vi "Test Serializer.Text.issue5.vi"(8 "error in (no error)":errorcluster) -> (0 "error out":errorcluster)   [LabVIEW 2013]
uses:
  source/Serializer.PlainText/Serializer.PlainText.lvclass
  <vilib>/addons/_JKI Toolkits/Caraya/classes/Assert/Assert Not Error.vi
  <vilib>/addons/_JKI Toolkits/Caraya/classes/Assert/Assert Equal Value and Type_Variant.vi
  <vilib>/addons/_JKI Toolkits/Caraya/classes/Assert/Assert.lvclass
  source/Serializer/Serializer.lvclass
  <vilib>/addons/_JKI Toolkits/Caraya/classes/Test/Test.lvclass
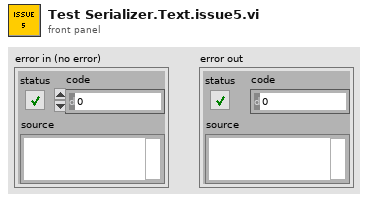
[diagram p1: front panel]
types:
  T1 = cluster{"String":string, "Cluster Array":cluster{"String":string, "Number":i16}[]}
  T2 = cluster{"String":string, "Cluster 2":cluster{"String":string, "Number":i16}}[]
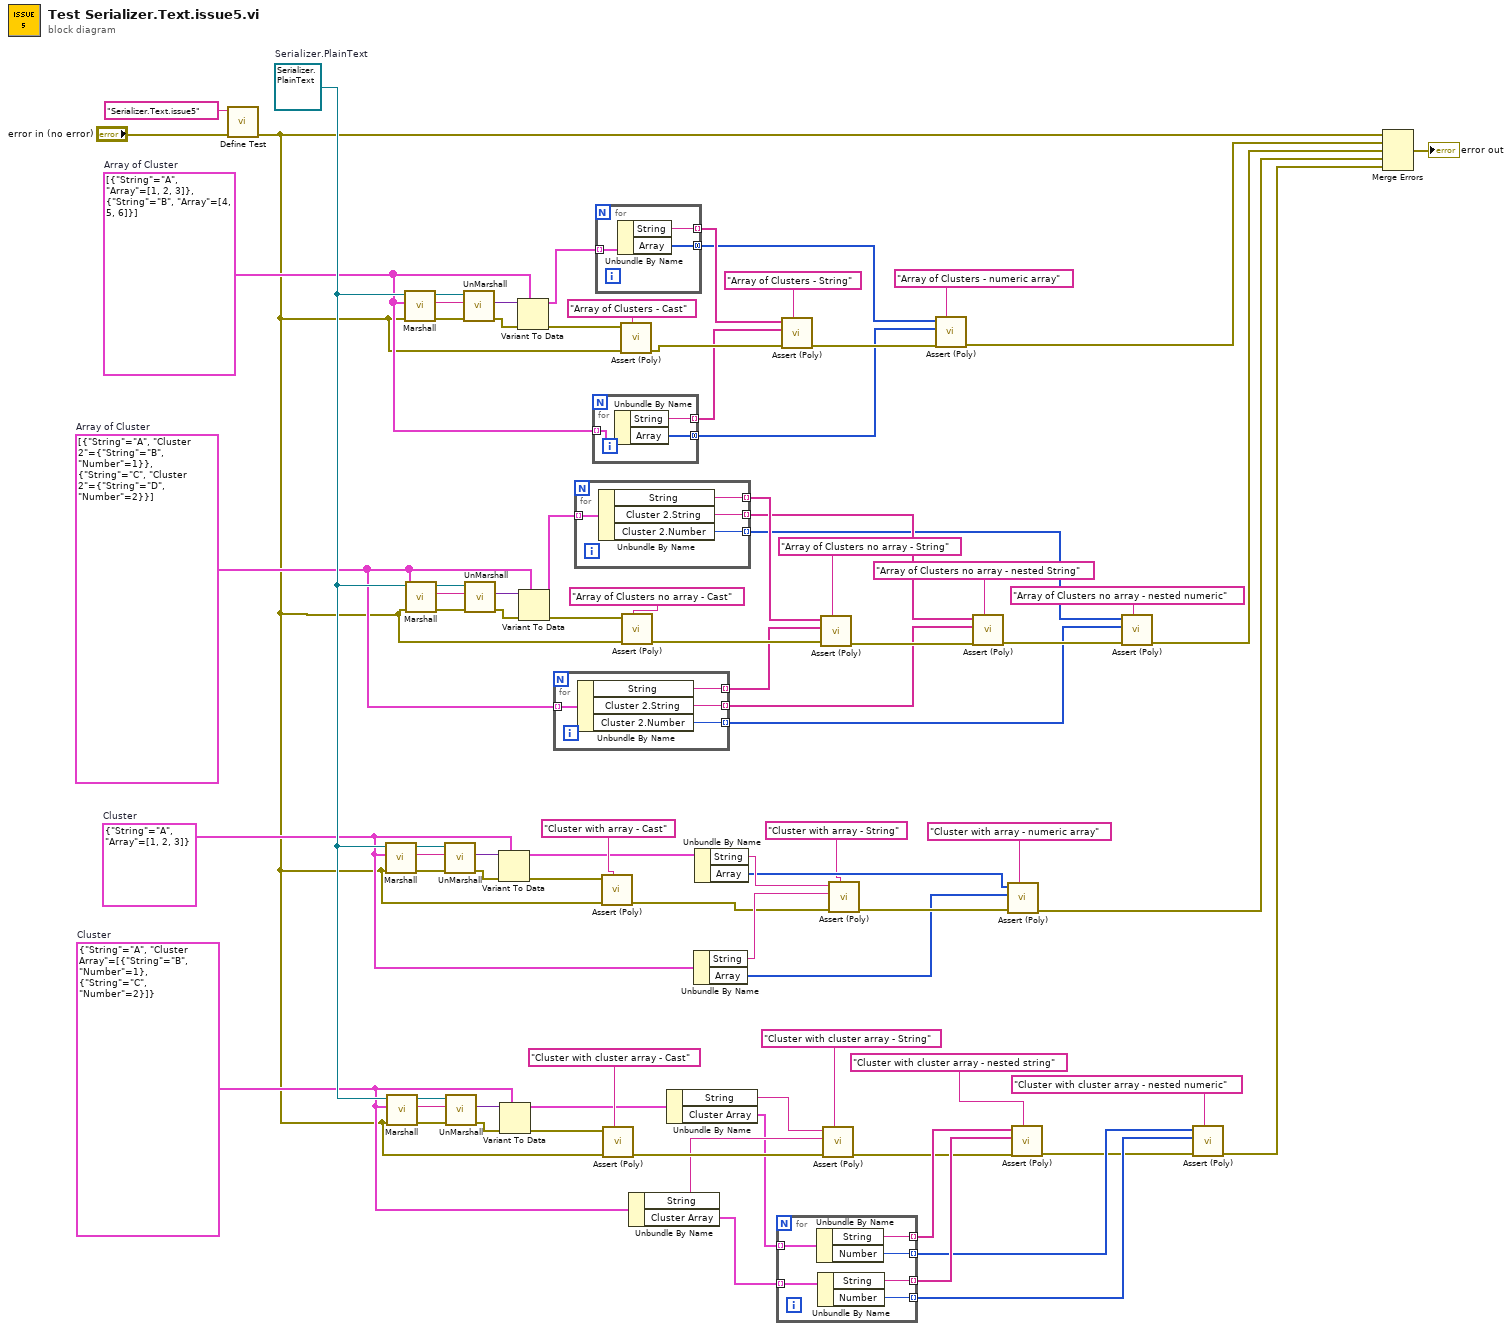
[diagram p0: block diagram]
diagram:
  w18 = T1 {"String"="A", "Cluster Array"=[{"String"="B", "Number"=1}, {"String"="C", "Number"=2}]}  # Cluster
  w31 = cluster{"String":string, "Array":i16[]} {"String"="A", "Array"=[1, 2, 3]}  # Cluster
  w3 = T2 [{"String"="A", "Cluster 2"={"String"="B", "Number"=1}}, {"String"="C", "Cluster 2"={"String"="D", "Number"=2}}]  # Array of Cluster
  w4 = cluster{"String":string, "Array":i16[]}[] [{"String"="A", "Array"=[1, 2, 3]}, {"String"="B", "Array"=[4, 5, 6]}]  # Array of Cluster
  w57 = refnum<class "Serializer.PlainText.lvclass"> refnum  # Serializer.PlainText
  n1 = call <vilib>:"Define Test.vi"("error in (no error)"="error in (no error)", "Label (VI Title)"="Serializer.Text.issue5") -> ("error out"=w1:errorcluster)  [unwired: 9 in]
  n2 = call "Marshall.vi"("error in (no error)"=w1, "Variant"=w31, "Serializer in"=w57) -> ("error out"=w70:errorcluster, "String"=w72:string, "Serializer out"=w71:refnum<class "Serializer.PlainText.lvclass">)  [unwired: 6 in]
  n3 = call "Marshall.vi"("error in (no error)"=w1, "Variant"=w18, "Serializer in"=w57) -> ("error out"=w61:errorcluster, "String"=w59:string, "Serializer out"=w60:refnum<class "Serializer.PlainText.lvclass">)  [unwired: 6 in]
  n4 = call "Marshall.vi"("error in (no error)"=w1, "Variant"=w4, "Serializer in"=w57) -> ("error out"=w82:errorcluster, "String"=w84:string, "Serializer out"=w83:refnum<class "Serializer.PlainText.lvclass">)  [unwired: 6 in]
  n5 = call "Marshall.vi"("error in (no error)"=w1, "Variant"=w3, "Serializer in"=w57) -> ("error out"=w77:errorcluster, "String"=w75:string, "Serializer out"=w76:refnum<class "Serializer.PlainText.lvclass">)  [unwired: 6 in]
  n6 = call "UnMarshall.vi"("error in (no error)"=w70, "String"=w72, "Serializer in"=w71) -> ("error out"=w65:errorcluster, "Variant"=w69:variant)  [unwired: 6 in, 1 out]
  n7 = call "UnMarshall.vi"("error in (no error)"=w61, "String"=w59, "Serializer in"=w60) -> ("error out"=w64:errorcluster, "Variant"=w62:variant)  [unwired: 6 in, 1 out]
  n8 = call "UnMarshall.vi"("error in (no error)"=w82, "String"=w84, "Serializer in"=w83) -> ("error out"=w67:errorcluster, "Variant"=w81:variant)  [unwired: 6 in, 1 out]
  n9 = call "UnMarshall.vi"("error in (no error)"=w77, "String"=w75, "Serializer in"=w76) -> ("error out"=w66:errorcluster, "Variant"=w78:variant)  [unwired: 6 in, 1 out]
  n10 = Variant To Data(error in=w65, type=w31, Variant=w69) -> (data=w32:cluster{"String":string, "Array":i16[]}, error out=w68:errorcluster)
  n11 = Variant To Data(error in=w64, type=w18, Variant=w62) -> (data=w19:T1, error out=w63:errorcluster)
  n12 = Variant To Data(error in=w67, type=w4, Variant=w81) -> (data=w51:cluster{"String":string, "Array":i16[]}[], error out=w80:errorcluster)
  n13 = Variant To Data(error in=w66, type=w3, Variant=w78) -> (data=w50:T2, error out=w79:errorcluster)
  n14 = for {
    tunnel: w3 -> [w91] mode=indexing
    tunnel: [w90] -> w37 mode=indexing
    tunnel: [w89] -> w35 mode=indexing
    tunnel: [w88] -> w33 mode=indexing
    n15 = Unbundle By Name(w91) -> ("String"=w90:string, "Cluster 2.String"=w89:string, "Cluster 2.Number"=w88:i16)
  }
  n16 = for {
    tunnel: w50 -> [w95] mode=indexing
    tunnel: [w94] -> w38 mode=indexing
    tunnel: [w93] -> w36 mode=indexing
    tunnel: [w92] -> w34 mode=indexing
    n17 = Unbundle By Name(w95) -> ("String"=w94:string, "Cluster 2.String"=w93:string, "Cluster 2.Number"=w92:i16)
  }
  n18 = for {
    tunnel: [w98] -> w47 mode=concatenating
    tunnel: [w97] -> w48 mode=indexing
    tunnel: w4 -> [w96] mode=indexing
    n19 = Unbundle By Name(w96) -> ("String"=w97:string, "Array"=w98:i16[])
  }
  n20 = for {
    tunnel: w51 -> [w101] mode=indexing
    tunnel: [w100] -> w46 mode=concatenating
    tunnel: [w99] -> w49 mode=indexing
    n21 = Unbundle By Name(w101) -> ("String"=w99:string, "Array"=w100:i16[])
  }
  n22 = call-poly <vilib>:"Assert (Poly).vi"("Label"="Cluster with array - Cast", "error in (no error)"=w1, "Not Error?"=w68) -> ("error out"=w28:errorcluster)  [unwired: 8 in]
  n23 = call-poly <vilib>:"Assert (Poly).vi"("Label"="Cluster with cluster array - Cast", "error in (no error)"=w1, "Not Error?"=w63) -> ("error out"=w21:errorcluster)  [unwired: 8 in]
  n24 = call-poly <vilib>:"Assert (Poly).vi"("Label"="Array of Clusters - Cast", "error in (no error)"=w1, "Not Error?"=w80) -> ("error out"=w56:errorcluster)  [unwired: 8 in]
  n25 = call-poly <vilib>:"Assert (Poly).vi"("Label"="Array of Clusters no array - Cast", "error in (no error)"=w1, "Not Error?"=w79) -> ("error out"=w42:errorcluster)  [unwired: 8 in]
  n26 = Unbundle By Name(w18) -> ("String"=w14:string, "Cluster Array"=w13:cluster{"String":string, "Number":i16}[])
  n27 = Unbundle By Name(w19) -> ("String"=w15:string, "Cluster Array"=w12:cluster{"String":string, "Number":i16}[])
  n28 = Unbundle By Name(w31) -> ("String"=w29:string, "Array"=w25:i16[])
  n29 = Unbundle By Name(w32) -> ("String"=w30:string, "Array"=w26:i16[])
  n30 = for {
    tunnel: w13 -> [w106] mode=indexing
    tunnel: w12 -> [w107] mode=indexing
    tunnel: [w105] -> w11 mode=indexing
    tunnel: [w104] -> w9 mode=indexing
    tunnel: [w103] -> w10 mode=indexing
    tunnel: [w102] -> w8 mode=indexing
    n31 = Unbundle By Name(w107) -> ("String"=w105:string, "Number"=w104:i16)
    n32 = Unbundle By Name(w106) -> ("String"=w103:string, "Number"=w102:i16)
  }
  n33 = call-poly <vilib>:"Assert (Poly).vi"("Label"="Array of Clusters - String", "error in (no error)"=w56, "Y"=w48, "X"=w49) -> ("error out"=w55:errorcluster)  [unwired: 7 in]
  n34 = call-poly <vilib>:"Assert (Poly).vi"("Label"="Array of Clusters no array - String", "error in (no error)"=w42, "Y"=w37, "X"=w38) -> ("error out"=w41:errorcluster)  [unwired: 7 in]
  n35 = call-poly <vilib>:"Assert (Poly).vi"("Label"="Cluster with cluster array - String", "error in (no error)"=w21, "Y"=w14, "X"=w15) -> ("error out"=w7:errorcluster)  [unwired: 7 in]
  n36 = call-poly <vilib>:"Assert (Poly).vi"("Label"="Cluster with array - String", "error in (no error)"=w28, "Y"=w29, "X"=w30) -> ("error out"=w27:errorcluster)  [unwired: 7 in]
  n37 = call-poly <vilib>:"Assert (Poly).vi"("Label"="Array of Clusters - numeric array", "error in (no error)"=w55, "Y"=w47, "X"=w46) -> ("error out"=w54:errorcluster)  [unwired: 7 in]
  n38 = call-poly <vilib>:"Assert (Poly).vi"("Label"="Array of Clusters no array - nested String", "error in (no error)"=w41, "Y"=w35, "X"=w36) -> ("error out"=w40:errorcluster)  [unwired: 7 in]
  n39 = call-poly <vilib>:"Assert (Poly).vi"("Label"="Cluster with array - numeric array", "error in (no error)"=w27, "Y"=w25, "X"=w26) -> ("error out"=w24:errorcluster)  [unwired: 7 in]
  n40 = call-poly <vilib>:"Assert (Poly).vi"("Label"="Cluster with cluster array - nested string", "error in (no error)"=w7, "Y"=w10, "X"=w11) -> ("error out"=w6:errorcluster)  [unwired: 7 in]
  n41 = call-poly <vilib>:"Assert (Poly).vi"("Label"="Array of Clusters no array - nested numeric", "error in (no error)"=w40, "Y"=w33, "X"=w34) -> ("error out"=w39:errorcluster)  [unwired: 7 in]
  n42 = call-poly <vilib>:"Assert (Poly).vi"("Label"="Cluster with cluster array - nested numeric", "error in (no error)"=w6, "Y"=w8, "X"=w9) -> ("error out"=w5:errorcluster)  [unwired: 7 in]
  n43 = Merge Errors(w1, w54, w39, w24, w5) -> (→"error out":errorcluster)
